vi "test5.vi"() -> ()   [LabVIEW 2016]
panel:
  out "数值 3":dbl
  in  "数值 2":dbl
  in  "数值":dbl
  # "商与余数"
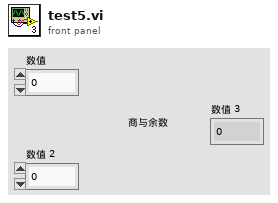
[diagram p1: front panel]
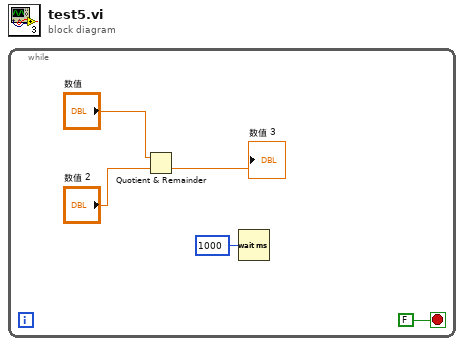
[diagram p0: block diagram]
diagram:
  n1 = while {
    stop <- FALSE stop-if-true
    n2 = Quotient & Remainder(x="数值", y="数值 2") -> (floor(x/y)=→"数值 3":dbl)  [unwired: 1 out]
    n3 = Wait (ms)(milliseconds to wait=u32 1000 ("等待时间（毫秒）")) -> ()  [unwired: 1 out]
  }
